vi "Configure Arbitrary Sequence [SEQ].vi"(5 "offset (0.00 V)":dbl[unit] format="%.4f", 7 "gain (1.00)":dbl=1.0 format="%.4f", 8 "error in (no error)":errorcluster, 9 "sequence handle (0)":i32, 10 "channel name (\"CHANNEL1\")":string="CHANNEL1", 11 "CS++Fgen in":refnum<class "CS++Fgen.lvclass">) -> (0 "error out":errorcluster, 3 "CS++Fgen out":refnum<class "CS++Fgen.lvclass">)   [LabVIEW 2016, in "CS++Fgen.lvlib" / "CS++Fgen.lvclass"]
doc: "This VI configures the properties of the function generator that affect arbitrary sequence generation. These properties are the arbitrary sequence handle, gain, and offset.\n\nNotes:\n\n(1) This VI is part of the IviFgenArbSeq [SEQ] extension group."
uses:
  CS++Fgen.lvclass
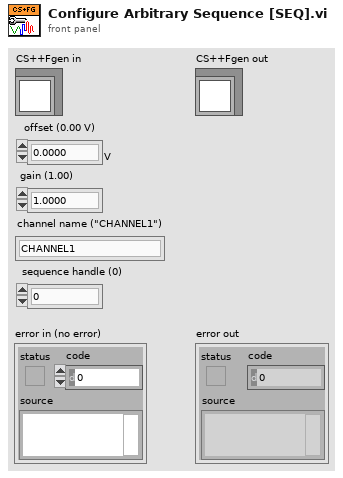
[diagram p1: front panel]
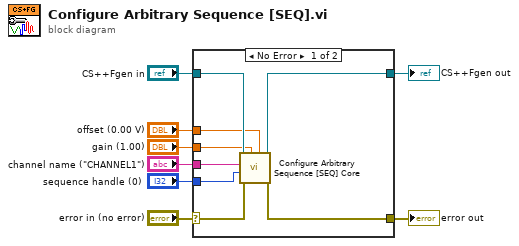
[diagram p0: block diagram]
diagram:
  n1 = case shown="No Error" "error in (no error)" {
    selector: "error in (no error)" -> [w14 w18]
    tunnel: [w13 w18] -> w7
    tunnel: [w15 w17] -> w5
    tunnel: "CS++Fgen in" -> [w16 w17]
    tunnel: "channel name (\"CHANNEL1\")" -> [w12 _]
    tunnel: "offset (0.00 V)" -> [w9 _]
    tunnel: "gain (1.00)" -> [w10 _]
    tunnel: "sequence handle (0)" -> [w11 _]
    frame No Error {
      n2 = call-dynamic "Configure Arbitrary Sequence [SEQ] Core.vi"("offset (0.00 V)"=w9, "gain (1.00)"=w10, "error in (no error)"=w14, "sequence handle (0)"=w11, "channel name (\"CHANNEL1\")"=w12, "CS++Fgen in"=w16) -> ("error out"=w13:errorcluster, "CS++Fgen out"=w15:refnum<class "CS++Fgen.lvclass">)  [unwired: 4 in]
    }
    frame Error {
    }
  }
  "error out" <- w7
  "CS++Fgen out" <- w5
